vi "PassThru.vi"(8 "error in (no error)":errorcluster, 9 "timeout ms (1000)":i32=1000, 10 "Cmd":cluster{"cmd":u8[], "require response?":bool}={"cmd"=[], "require response?"=TRUE}, 11 "Connection Info":T1) -> (0 "error out":errorcluster, 2 "Resp":T3, 3 "Connection Info":T1)   [LabVIEW 2015, in "Diagnostics Host Automation API.lvlib"]
uses:
  Diagnostics Host Automation API.lvlib
  <userlib>/STM/TCP/stm_TCP Connection Info.ctl
  <userlib>/STM/_SubVIs/stm_MetaDataElement.ctl
  Shared/Types/RequestResponse Data Cluster.ctl
  <userlib>/STM/TCP/stm_TCP Write Options.ctl
  <userlib>/STM/TCP/STM Write Message (TCP).vi
  <userlib>/STM/TCP/STM Read Message (TCP).vi
  Shared/Diagnostics Addon Shared.lvlib
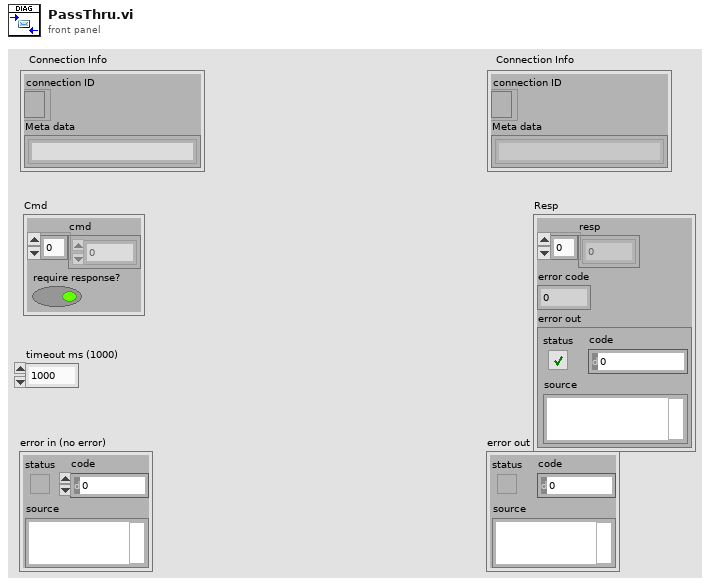
[diagram p1: front panel]
types:
  T1 = typedef "stm_TCP Connection Info.ctl" = cluster{"connection ID":refnum<k5>, "Meta data":T2[]}
  T2 = typedef "stm_MetaDataElement.ctl" = string
  T3 = cluster{"resp":u8[], "error code":u8, "error out":errorcluster}
  T4 = typedef "stm_TCP Write Options.ctl" = cluster{"Ignore Timeout Error":bool, "timeout ms (1000)":i32}
  T5 = typedef "Diagnostics Addon Shared.lvlib/RequestResponse Data Cluster.ctl" = cluster{"Timeout":i32, "data":string}
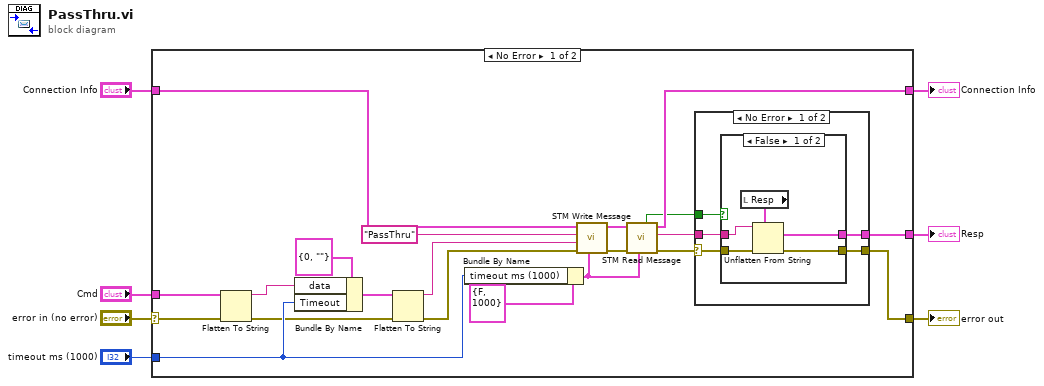
[diagram p0: block diagram]
diagram:
  n1 = case shown="No Error" "error in (no error)" {
    selector: "error in (no error)" -> [w12 w42]
    tunnel: "Connection Info" -> [w28 w41]
    tunnel: [w25 w41] -> w6
    tunnel: [w15 w42] -> w5
    tunnel: "timeout ms (1000)" -> [w13 _]
    tunnel: "Cmd" -> [w9 _]
    tunnel: [w8 _] -> w1
    frame No Error {
      n2 = Flatten To String(anything=w9, error in (no error)=w12) -> (data string=w10:string, error out=w11:errorcluster)  [unwired: 2 in, 1 out]
      n3 = Bundle By Name(cluster=T5 {"Timeout"=0, "data"=""}, "data"=w10, "Timeout"=w13) -> (w22:T5)
      n4 = Flatten To String(anything=w22, error in (no error)=w11) -> (data string=w20:string, error out=w21:errorcluster)  [unwired: 2 in, 1 out]
      n5 = Bundle By Name(cluster=T4 {"Ignore Timeout Error"=FALSE, "timeout ms (1000)"=1000} ("Options"), "timeout ms (1000)"=w13) -> (w18:T4)
      n6 = call-poly <userlib>:"STM Write Message.vi"("Options"=w18, "error in (no error)"=w21, "Data"=w20, "Name"="PassThru", "Connection Info"=w28) -> ("error out"=w24:errorcluster, "Connection Info Out"=w26:T1)  [unwired: 5 in]
      n7 = call-poly <userlib>:"STM Read Message.vi"("Options"=w18, "error in"=w24, "Connection Info"=w26) -> ("error out"=w17:errorcluster, "data string"=w14:string, "Connection Info Out"=w25:T1, "Timed Out?"=w16:bool)  [unwired: 3 in, 2 out]
      n8 = case shown="No Error" w17 {
        selector: w17 -> [w31 w40]
        tunnel: w16 -> [w33 _]
        tunnel: [w32 w40] -> w15
        tunnel: w14 -> [w30 _]
        tunnel: [w29 _] -> w8
        frame No Error {
          n9 = case shown="False" w33 {
            tunnel: [w35 w39] -> w32
            tunnel: w31 -> [w36 w39]
            tunnel: w30 -> [w37 _]
            tunnel: [w34 _] -> w29
            frame False {
              n10 = local read "Resp"() -> (w38:T3)
              n11 = Unflatten From String(type=w38, binary string=w37, error in (no error)=w36) -> (value=w34:T3, error out=w35:errorcluster)  [unwired: 2 in, 1 out]
            }
            frame True {
            }
          }
        }
        frame Error {
        }
      }
    }
    frame Error {
    }
  }
  "Connection Info" <- w6
  "error out" <- w5
  "Resp" <- w1
